vi "SyncOutputs.vi"(8 "error in (no error)":errorcluster, 10 "fpMgr in":refnum<class "VIProviderShellHelper.lvclass">, 11 "Shell in":refnum<class "VIProviderShellHelper.lvclass">) -> (0 "error out":errorcluster, 2 "fpMgr out":refnum<class "VIProviderShellHelper.lvclass">, 3 "Shell out":refnum<class "VIProviderShellHelper.lvclass">)   [LabVIEW 2019, in "LabVIEW-ProviderShell.lvlib" / "VIProviderShellHelper.lvclass"]
uses:
  VIProviderShellHelper.lvclass
  VIProviderShellHelper.lvclass/VIProviderShellHelper.ctl
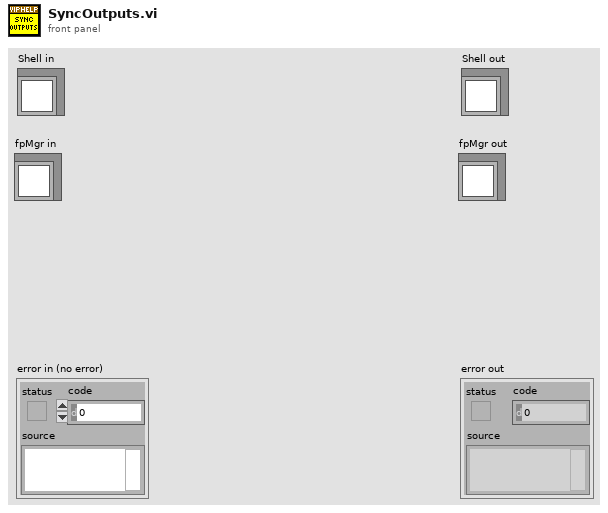
[diagram p1: front panel]
types:
  T1 = typedef "LabVIEW-ProviderShell.lvlib/VIProviderShellHelper.lvclass/def-ConnectorInfo.ctl" = cluster{"Value":variant, "Label.Text":string, "error":errorcluster, "DatatypeDescription":string, "Indicator":bool}
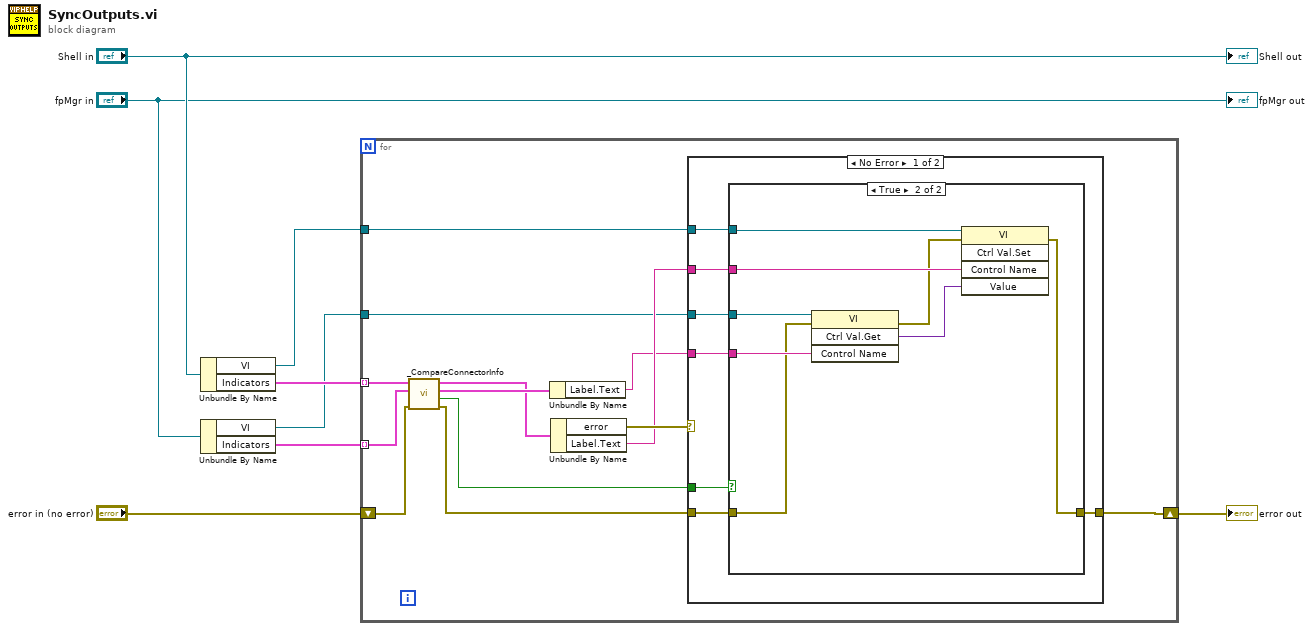
[diagram p0: block diagram]
diagram:
  n1 = Unbundle By Name("Shell in") -> ("VI"=w2:refnum<vi>, "Indicators"=w6:T1[])
  n2 = Unbundle By Name("fpMgr in") -> ("VI"=w1:refnum<vi>, "Indicators"=w5:T1[])
  n3 = for {
    tunnel: w6 -> [w19] mode=indexing
    tunnel: w5 -> [w18] mode=indexing
    shift-right: [w21] -> w3
    shift-left: "error in (no error)" -> [w16]
    tunnel: w2 -> [w12]
    tunnel: w1 -> [w9]
    n4 = call "_CompareConnectorInfo.vi"("error in (no error)"=w16, 10:"Cluster"=w18, 11:"Cluster"=w19) -> ("error out"=w15:errorcluster, "Matched"=w17:bool, 2:"Cluster"=w14:T1, 3:"Cluster"=w13:T1)  [unwired: 5 in]
    n5 = Unbundle By Name(w14) -> ("Label.Text"=w10:string)
    n6 = Unbundle By Name(w13) -> ("error"=w20:errorcluster, "Label.Text"=w11:string)
    n7 = case shown="No Error" w20 {
      tunnel: w15 -> [w28 w38]
      tunnel: [w27 w38] -> w21
      tunnel: w17 -> [w24 _]
      tunnel: w12 -> [w26 _]
      tunnel: w11 -> [w25 _]
      tunnel: w10 -> [w23 _]
      tunnel: w9 -> [w22 _]
      frame No Error {
        n8 = case shown="True" w24 {
          tunnel: w28 -> [w29 w31]
          tunnel: [w29 w35] -> w27
          tunnel: w26 -> [_ w37]
          tunnel: w25 -> [_ w36]
          tunnel: w23 -> [_ w34]
          tunnel: w22 -> [_ w32]
          frame False {
          }
          frame True {
            n9 = invoke class="VI" method="Ctrl Val.Get"(reference=w32, error in=w31, "Control Name"=w34) -> (error out=w30:errorcluster, "Get Control Value Variant"=w33:variant)  [unwired: 1 in, 2 out]
            n10 = invoke class="VI" method="Ctrl Val.Set"(reference=w37, error in=w30, "Control Name"=w36, "Value"=w33) -> (error out=w35:errorcluster)  [unwired: 1 in, 4 out]
          }
        }
      }
      frame Error {
      }
    }
  }
  "error out" <- w3
  "Shell out" <- "Shell in"
  "fpMgr out" <- "fpMgr in"
